vi "ReadGraphSettings.vi"(8 "Error In":errorcluster, 11 "VI in":refnum<vi>) -> (0 "Error Out":errorcluster)   [LabVIEW 2018]
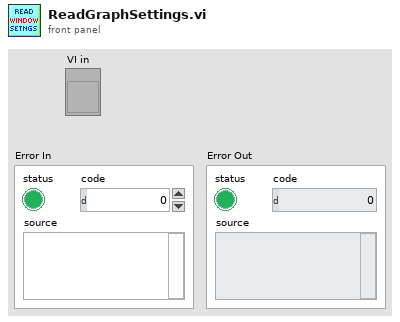
[diagram p1: front panel]
types:
  T1 = enum16{"open", "replace", "create", "open or create", "replace or create", "replace or create with confirmation"}
  T2 = enum32{"Invalid", "Standard", "Closed", "Hidden", "Minimized", "Maximized"}
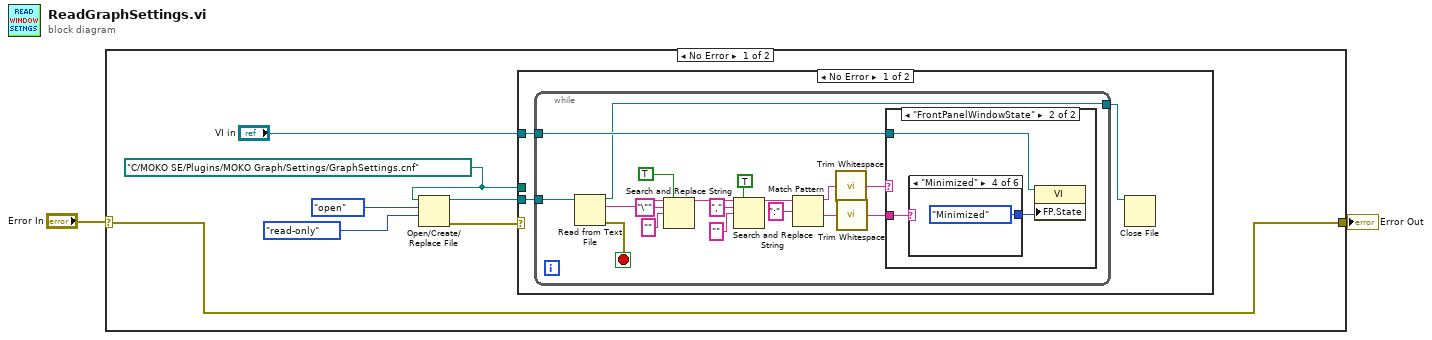
[diagram p0: block diagram]
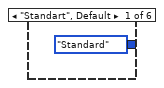
[diagram p3: hidden frame]
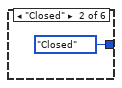
[diagram p4: hidden frame]
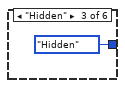
[diagram p5: hidden frame]
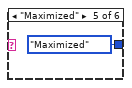
[diagram p6: hidden frame]
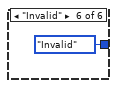
[diagram p7: hidden frame]
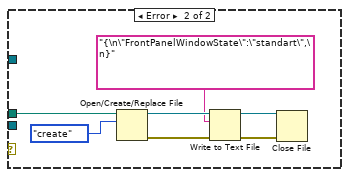
[diagram p8: hidden frame]
diagram:
  n1 = case shown="No Error" "Error In" {
    selector: "Error In" -> [w6 w47]
    tunnel: [w6 w47] -> w1
    frame No Error {
      w4 = path "C:/MOKO SE/Plugins/MOKO Graph/Settings/GraphSettings.cnf" ("file path (use dialog)")
      n2 = Open/Create/Replace File(file path (use dialog)=w4, operation (0:open)=T1."open", access (0:read/write)=enum16{"read/write", "read-only", "write-only"}."read-only") -> (refnum out=w3:refnum<file>, error out=w5:errorcluster)  [unwired: 3 in, 1 out]
      n3 = case shown="No Error" w5 {
        tunnel: "VI in" -> [w12 _]
        tunnel: w4 -> [_ w46]
        tunnel: w3 -> [w11 _]
        frame No Error {
          n4 = while {
            tunnel: w12 -> [w29]
            tunnel: w11 -> [w14]
            tunnel: [w13] -> w10
            stop <- w30 stop-if-true
            n5 = Read from Text File(file (use dialog)=w14) -> (refnum out=w13:refnum<file>, text=w26:string, error out=w30:errorcluster)  [unwired: 3 in, 1 out]
            n6 = Search and Replace String(replace all?=TRUE ("replace all? (F)"), input string=w26, search string="\"", replace string="" ("replace string (\"\")")) -> (result string=w22:string)  [unwired: 4 in, 3 out]
            n7 = Search and Replace String(replace all?=TRUE ("replace all? (F)"), input string=w22, search string=",", replace string="" ("replace string (\"\")")) -> (result string=w18:string)  [unwired: 4 in, 3 out]
            n8 = Match Pattern(string=w18, regular expression=":") -> (before substring=w28:string, after substring=w27:string)  [unwired: 1 in, 2 out]
            n9 = call <vilib>:"Trim Whitespace.vi"("string"=w28) -> ("trimmed string"=w16:string)  [unwired: 1 in]
            n10 = call <vilib>:"Trim Whitespace.vi"("string"=w27) -> ("trimmed string"=w15:string)  [unwired: 1 in]
            n11 = case shown="\"FrontPanelWindowState\"" w16 {
              tunnel: w29 -> [_ w33]
              tunnel: w15 -> [_ w32]
              frame "False", Default {
              }
              frame "FrontPanelWindowState" {
                n12 = case shown="\"Minimized\"" w32 {
                  tunnel: [T2."Standard" ("Front Panel Window:State") T2."Closed" ("Front Panel Window:State") T2."Hidden" ("Front Panel Window:State") T2."Minimized" ("Front Panel Window:State") T2."Maximized" ("Front Panel Window:State") T2."Invalid" ("Front Panel Window:State")] -> w31
                  frame "Standart", Default {
                  }
                  frame "Closed" {
                  }
                  frame "Hidden" {
                  }
                  frame "Minimized" {
                  }
                  frame "Maximized" {
                  }
                  frame "Invalid" {
                  }
                }
                n13 = property class="VI"(reference=w33, "FP.State"=w31) -> ()  [unwired: 1 in, 2 out]
              }
            }
          }
          n14 = Close File(refnum=w10) -> ()  [unwired: 1 in, 2 out]
        }
        frame Error {
          n15 = Open/Create/Replace File(file path (use dialog)=w46, operation (0:open)=T1."create") -> (refnum out=w44:refnum<file>, error out=w41:errorcluster)  [unwired: 4 in, 1 out]
          n16 = Write to Text File(file (use dialog)=w44, text="{\n\"FrontPanelWindowState\":\"standart\",\n}", error in=w41) -> (refnum out=w42:refnum<file>, error out=w40:errorcluster)  [unwired: 1 in, 1 out]
          n17 = Close File(refnum=w42, error in=w40) -> ()  [unwired: 2 out]
        }
      }
    }
    frame Error {
    }
  }
  "Error Out" <- w1
